vi "Color Scaler.vi"(1 "Upper numberlimit (default 30)":dbl, 2 "Lower numberlimit (default 18)":dbl, 3 "Upper colourlimit":u32(colorbox), 4 "Input":dbl, 5 "Boolean (False =Temp;True=hum)":bool, 6 "Lower colourlimit":u32(colorbox)) -> (0 "Output Color":u32(colorbox))   [LabVIEW 2021]
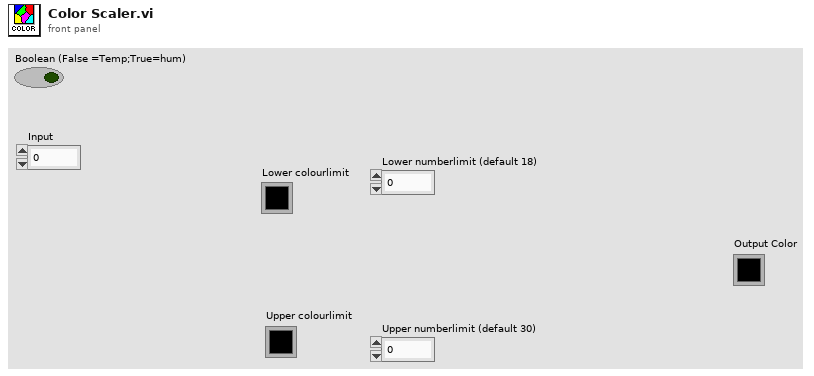
[diagram p1: front panel]
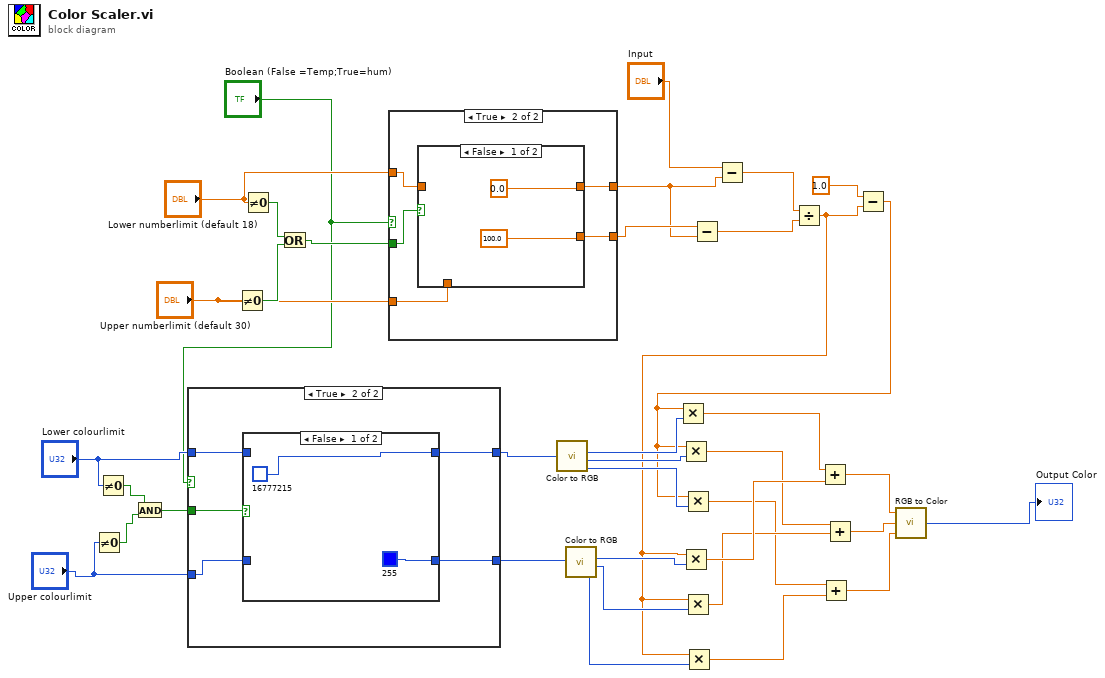
[diagram p0: block diagram]
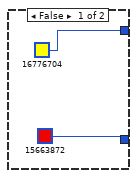
[diagram p3: hidden frame]
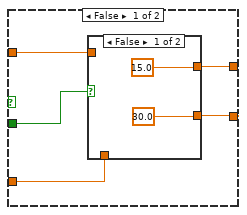
[diagram p5: hidden frame]
diagram:
  n1 = Not Equal To 0?(x="Upper colourlimit") -> (x != 0?=w25:bool)
  n2 = Not Equal To 0?(x="Lower colourlimit") -> (x != 0?=w24:bool)
  n3 = And(x=w24, y=w25) -> (x .and. y?=w1:bool)
  n4 = case shown="True" "Boolean (False =Temp;True=hum)" {
    tunnel: "Lower colourlimit" -> [w39 w48]
    tunnel: "Upper colourlimit" -> [w38 w47]
    tunnel: [w42 w50] -> w22
    tunnel: [w41 w49] -> w21
    tunnel: w1 -> [w40 w51]
    frame False {
      n5 = case shown="True" w40 {
        tunnel: [u32 16776704 ("Upper colourlimit") w46] -> w42
        tunnel: [u32 15663872 ("Upper colourlimit") w45] -> w41
        tunnel: w39 -> [_ w46]
        tunnel: w38 -> [_ w45]
        frame False {
        }
        frame True {
        }
      }
    }
    frame True {
      n6 = case shown="False" w51 {
        tunnel: [u32 16777215 ("Upper colourlimit") w55] -> w50
        tunnel: [u32 255 ("Upper colourlimit") w54] -> w49
        tunnel: w48 -> [_ w55]
        tunnel: w47 -> [_ w54]
        frame False {
        }
        frame True {
        }
      }
    }
  }
  n7 = Not Equal To 0?(x="Upper numberlimit (default 30)") -> (x != 0?=w35:bool)
  n8 = Not Equal To 0?(x="Lower numberlimit (default 18)") -> (x != 0?=w36:bool)
  n9 = Or(x=w36, y=w35) -> (x .or. y?=w37:bool)
  n10 = case shown="True" "Boolean (False =Temp;True=hum)" {
    tunnel: w37 -> [w60 w67]
    tunnel: [w59 w69] -> w28
    tunnel: [w58 w68] -> w29
    tunnel: "Lower numberlimit (default 18)" -> [w57 w66]
    tunnel: "Upper numberlimit (default 30)" -> [w56 w65]
    frame False {
      n11 = case shown="False" w60 {
        tunnel: [15.0 w64] -> w59
        tunnel: [30.0 w63] -> w58
        tunnel: w57 -> [_ w64]
        tunnel: w56 -> [_ w63]
        frame False {
        }
        frame True {
        }
      }
    }
    frame True {
      n12 = case shown="False" w67 {
        tunnel: [0.0 ("Lower numberlimit") w73] -> w69
        tunnel: [100.0 ("Upper numberlimit") w72] -> w68
        tunnel: w66 -> [_ w73]
        tunnel: w65 -> [_ w72]
        frame False {
        }
        frame True {
        }
      }
    }
  }
  n13 = call <vilib>:"Color to RGB.vi"("Color"=w22) -> ("R"=w20:u8, "G"=w19:u8, "B"=w18:u8)  [unwired: 1 out]
  n14 = call <vilib>:"Color to RGB.vi"("Color"=w21) -> ("R"=w17:u8, "G"=w16:u8, "B"=w15:u8)  [unwired: 1 out]
  n15 = Subtract(x=w29, y=w28) -> (x-y=w30:dbl)
  n16 = Subtract(x="Input", y=w28) -> (x-y=w31:dbl)
  n17 = Divide(x=w31, y=w30) -> (x/y=w14:dbl)
  n18 = Multiply(x=w14, y=w17) -> (x*y=w11:dbl)
  n19 = Multiply(x=w14, y=w16) -> (x*y=w9:dbl)
  n20 = Multiply(x=w14, y=w15) -> (x*y=w7:dbl)
  n21 = Subtract(x=1.0, y=w14) -> (x-y=w13:dbl)
  n22 = Multiply(x=w13, y=w20) -> (x*y=w12:dbl)
  n23 = Multiply(x=w13, y=w19) -> (x*y=w10:dbl)
  n24 = Multiply(x=w13, y=w18) -> (x*y=w8:dbl)
  n25 = Add(x=w12, y=w11) -> (x+y=w6:dbl)
  n26 = Add(x=w8, y=w7) -> (x+y=w4:dbl)
  n27 = Add(x=w10, y=w9) -> (x+y=w5:dbl)
  n28 = call <vilib>:"RGB to Color.vi"("B"=w4, "G"=w5, "R"=w6) -> ("Color"=→"Output Color":u32)
